vi "FinnedHeatExchanger.vi"() -> ()   [LabVIEW 2017]
panel:
  out "Array":dbl[](array[numeric])
  in  "stop":bool
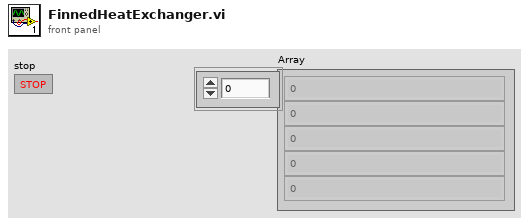
[diagram p1: front panel]
types:
  T1 = enum16{"open", "replace", "create", "open or create", "replace or create", "replace or create with confirmation"}
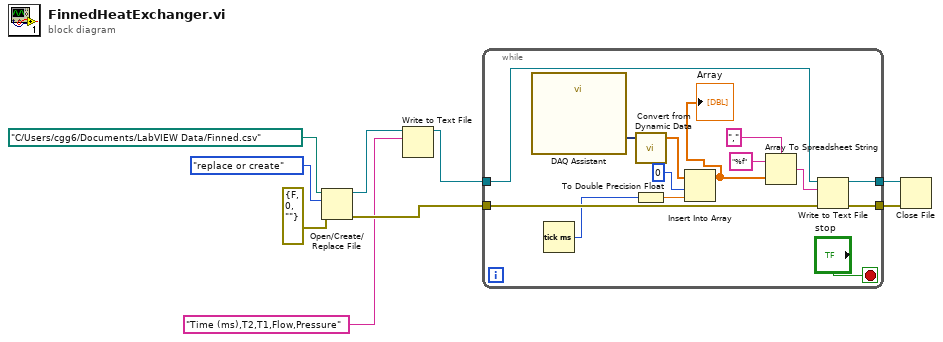
[diagram p0: block diagram]
diagram:
  n1 = Open/Create/Replace File(file path (use dialog)=path "C:/Users/cgg6/Documents/LabVIEW Data/Finned.csv", error in=errorcluster {"status"=FALSE, "code"=0, "source"=""}, operation (0:open)=T1."replace or create") -> (refnum out=w3:refnum<file>, error out=w6:errorcluster)  [unwired: 3 in, 1 out]
  n2 = Write to Text File(file (use dialog)=w3, text="Time (ms),T2,T1,Flow,Pressure") -> (refnum out=w2:refnum<file>)  [unwired: 2 in, 2 out]
  n3 = while {
    tunnel: w6 -> [w19]
    tunnel: [w18] -> w5
    tunnel: w2 -> [w17]
    tunnel: [w16] -> w4
    stop <- "stop" stop-if-true
    n4 = call "DAQ Assistant"() -> ("data"=w22:dynamicdata)  [unwired: 17 in, 2 out]
    n5 = Tick Count (ms)() -> (millisecond timer value=w10:u32)
    n6 = call "Convert from Dynamic Data"("Dynamic Data Type"=w22) -> ("Array"=w14:dbl[])  [unwired: 3 in]
    n7 = To Double Precision Float(number=w10) -> (double precision float=w13:dbl)
    n8 = Insert Into Array(array=w14, index=0, new element=w13) -> (w11:dbl[])
    "Array" <- w11
    n9 = Array To Spreadsheet String(delimiter (Tab)=",", array=w11, 3:"%f" ("format string")) -> (spreadsheet string=w15:string)
    n10 = Write to Text File(file (use dialog)=w17, text=w15, error in=w19) -> (refnum out=w16:refnum<file>, error out=w18:errorcluster)  [unwired: 1 in, 1 out]
  }
  n11 = Close File(refnum=w4, error in=w5) -> ()  [unwired: 2 out]
